vi "piezoWriteWriteSingleVolume.vi"(1 "scanDuration":dbl) -> ()   [LabVIEW 2017]
uses:
  <vilib>/DAQmx/write.llb/DAQmx Write (Analog 1D DBL 1Chan NSamp).vi
  globalDevices.vi
  globalUtilities.vi
  <vilib>/DAQmx/miscellaneous.llb/DAQmx Fill In Error Info.vi
panel:
  out "Waveform Graph":dbl[](graph)
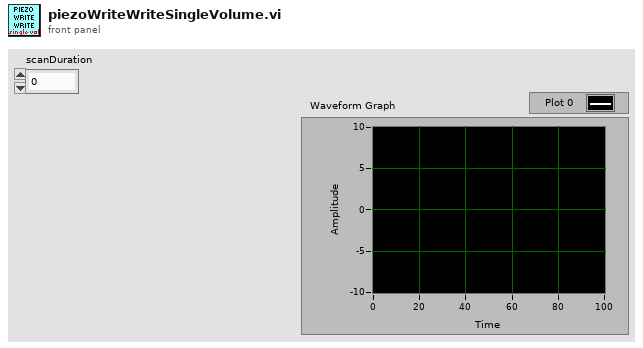
[diagram p1: front panel]
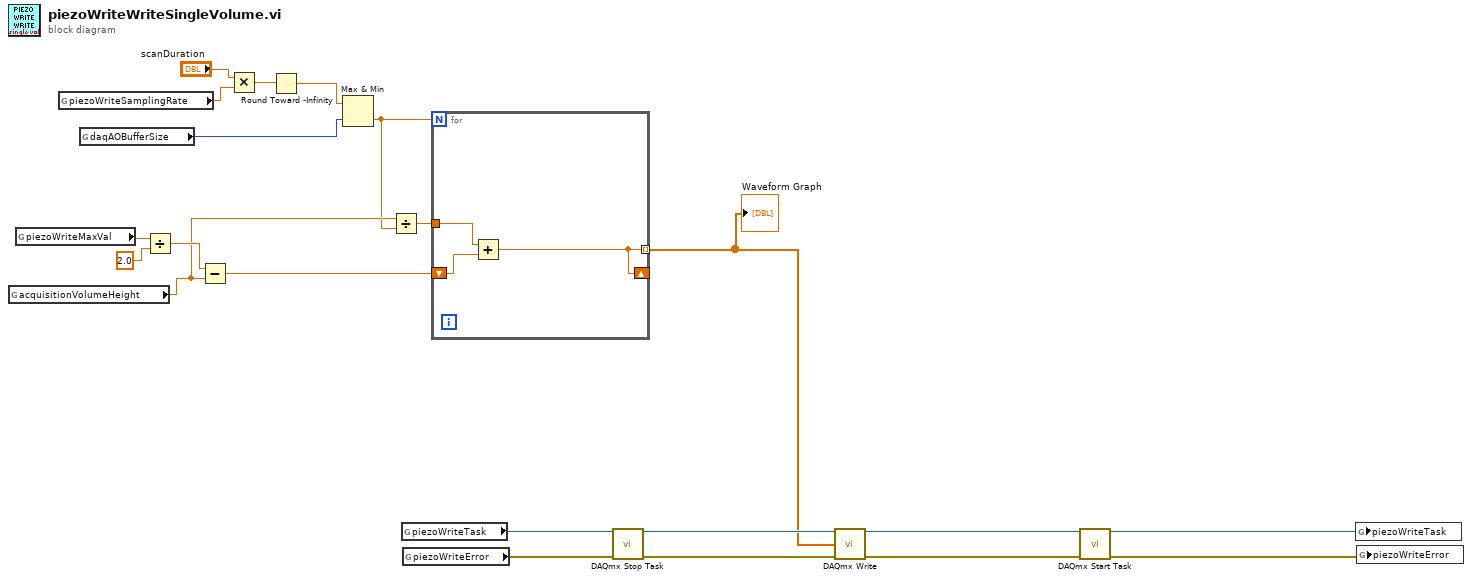
[diagram p0: block diagram]
diagram:
  n1 = global read "globalUtilities.vi" "acquisitionVolumeHeight"() -> (w5:dbl)
  n2 = global read "globalDevices.vi" "piezoWriteMaxVal"() -> (w13:dbl)
  n3 = global read "globalDevices.vi" "piezoWriteSamplingRate"() -> (w9:dbl)
  n4 = global read "globalDevices.vi" "daqAOBufferSize"() -> (w6:i32)
  n5 = Divide(x=w13, y=2.0) -> (x/y=w11:dbl)
  n6 = Subtract(x=w11, y=w5) -> (x-y=w2:dbl)
  n7 = Multiply(x="scanDuration", y=w9) -> (x*y=w8:dbl)
  n8 = Round Toward -Infinity(1:w8) -> (0:w7:dbl)
  n9 = Max & Min(x=w7, y=w6) -> (min(x,y)=w4:dbl)  [unwired: 1 out]
  n10 = Divide(x=w5, y=w4) -> (x/y=w3:dbl)
  n11 = global read "globalDevices.vi" "piezoWriteTask"() -> (w21:refnum<k21>)
  n12 = global read "globalDevices.vi" "piezoWriteError"() -> (w20:errorcluster)
  n13 = for {
    N: w4 -> [_]
    tunnel: w3 -> [w24]
    shift-right: [w22] -> _
    shift-left: w2 -> [w23]
    tunnel: [w22] -> w1 mode=indexing
    n14 = Add(x=w24, y=w23) -> (x+y=w22:dbl)
  }
  "Waveform Graph" <- w1
  n15 = call <vilib>:"DAQmx Stop Task.vi"("task/channels in"=w21, "error in"=w20) -> ("task out"=w19:refnum<k21>, "error out"=w18:errorcluster)  [unwired: 12 in]
  n16 = call-poly <vilib>:"DAQmx Write.vi"("task/channels in"=w19, "data"=w1, "error in"=w18) -> ("task out"=w15:refnum<k21>, "error out"=w14:errorcluster)  [unwired: 10 in, 1 out]
  n17 = call <vilib>:"DAQmx Start Task.vi"("task/channels in"=w15, "error in"=w14) -> ("task out"=w17:refnum<k21>, "error out"=w16:errorcluster)  [unwired: 12 in]
  n18 = global write "globalDevices.vi" "piezoWriteTask"(w17) -> ()
  n19 = global write "globalDevices.vi" "piezoWriteError"(w16) -> ()
